vi "Query SESR for Instrument Error.vi"(8 "error in (no error)":errorcluster {"code" format="%.0x"}, 11 "VISA session":refnum<visa-resource-name>) -> (0 "error out":errorcluster {"code" format="%.0x"}, 1 "Read SESR":T1, 3 "dup VISA session":refnum<visa-resource-name>)   [LabVIEW 2011]
doc: "Reads the instrument's IEEE-488.2 Standard Event Status Register. If the Standard Event indicates an instrument error occurred, error status in error out returns TRUE with the code and source indicating an instrument error.\n\nIf an instrument error occurs, send a query to retrieve instrument error details (e.g., send \"SYST:ERR?\" to retrieve error information).\n\nThe bits in the event register are cleared automatically after calling this VI.\n\nNotes: \n(1) Do not call this VI between a VISA Write sending an instrument query and the corresponding VISA Read that retrieves the response. Doing so likely results in a query error on your instrument.\n(2) If you want to read the Standard Event Status Register without updating the error out to reflect instrument errors, use the Query SESR.vi.\n(3) Calling this VI clears the contents of the Standard Event Status Register."
uses:
  Low Level/Standard Event Status Indicator.ctl
panel:
  # "standard event status register (SESR)"
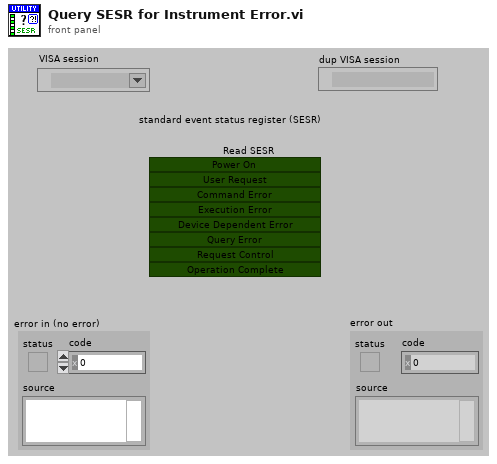
[diagram p1: front panel]
types:
  T1 = typedef "Standard Event Status Indicator.ctl" = cluster{"Operation Complete (1)":bool, "Request Control (2)":bool, "Query Error (4)":bool, "Device Dependent Error (8)":bool, "Execution Error (16)":bool, "Command Error (32)":bool, "User Request (64)":bool, "Power On (128)":bool}
  T2 = cluster{"[0]":bool, "[1]":bool, "[2]":bool, "[3]":bool, "[4]":bool, "[5]":bool, "[6]":bool, "[7]":bool}
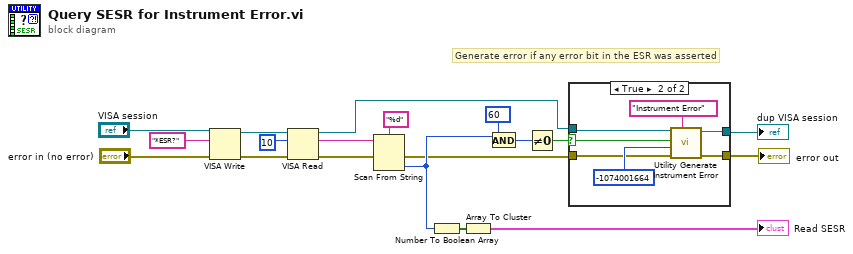
[diagram p0: block diagram]
diagram:
  # "Generate error if any error bit in the ESR was asserted"
  n1 = VISA Write(VISA resource name="VISA session", write buffer="*ESR?", error in (no error)="error in (no error)") -> (VISA resource name out=w12:refnum<visa-resource-name>, error out=w13:errorcluster)  [unwired: 1 out]
  n2 = VISA Read(VISA resource name=w12, byte count=10, error in (no error)=w13) -> (VISA resource name out=w1:refnum<visa-resource-name>, read buffer=w16:string, error out=w3:errorcluster)  [unwired: 1 out]
  n3 = Scan From String(format string="%d", input string=w16, error in=w3) -> (error out=w2:errorcluster, output 1=w4:i32)  [unwired: 2 in, 2 out]
  n4 = Number To Boolean Array(number=w4) -> (Boolean array=w17:bool[])
  n5 = Array To Cluster(array=w17) -> (cluster=→"Read SESR":T2)
  n6 = And(x=60, y=w4) -> (x .and. y?=w9:i32)
  n7 = Not Equal To 0?(x=w9) -> (x != 0?=w10:bool)
  n8 = case shown="True" w10 {
    selector: w10 -> [_ w25]
    tunnel: w1 -> [w21 w28]
    tunnel: w2 -> [w20 w22]
    tunnel: [w21 w27] -> w7
    tunnel: [w20 w26] -> w6
    frame False {
    }
    frame True {
      n9 = call "Utility Generate Instrument Error.vi"("Message"="Instrument Error", "error in (no error)"=w22, "Code (0)"=-1074001664 ("x"), "Is Warning? (F)"=w25, "VISA session"=w28) -> ("error out"=w26:errorcluster, "dup VISA session"=w27:refnum<visa-resource-name>)  [unwired: 5 in]
    }
  }
  "dup VISA session" <- w7
  "error out" <- w6
